vi "Log Error Event.vi"(8 "error in (no error)":errorcluster, 11 "Location":string) -> ()   [LabVIEW 2024, in "Sift Stream.lvlib" / "Sift Stream.lvclass"]
uses:
  Sift Stream.lvclass
  Log Event Types.ctl
  Sift Stream.lvclass/Sift Stream.ctl
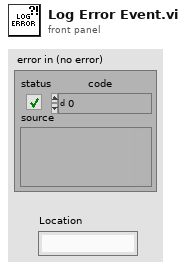
[diagram p1: front panel]
types:
  T1 = typedef "Sift Stream.lvlib/Sift Stream.lvclass/Log Event Types.ctl" = enum16{"INFO", "WARN", "ERROR"}
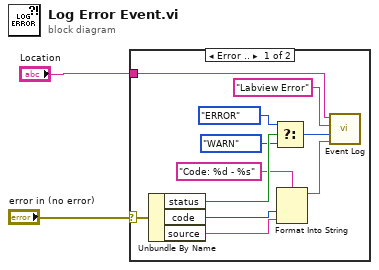
[diagram p0: block diagram]
diagram:
  n1 = case shown="Error .." "error in (no error)" {
    selector: "error in (no error)" -> [w4 _]
    tunnel: "Location" -> [w3 _]
    frame Error {
      n2 = Unbundle By Name(w4) -> ("status"=w13:bool, "code"=w7:i32, "source"=w6:string)
      n3 = Select(t=Log_Event_Types."ERROR" ("Log Event Types"), s=w13, f=Log_Event_Types."WARN" ("Log Event Types")) -> (s? t:f=w10:T1)
      n4 = Format Into String(format string="Code: %d - %s", w7, w6) -> (resulting string=w5:string)  [unwired: 2 in, 1 out]
      n5 = call "Event Log.vi"("Message"=w5, "Log Event Type"=w10, "Event Type"="Labview Error", "Location"=w3) -> ()  [unwired: 8 in]
    }
    frame No Error {
    }
  }
